vi "ImageInitRe.vi"(0 "Image in":refnum<class "Image.lvclass">, 11 "error in (no error)":errorcluster) -> (4 "Image out":refnum<class "Image.lvclass">, 15 "error out":errorcluster)   [LabVIEW 2012, in "Image.lvclass"]
uses:
  classes/Image.lvclass
  classes/Image.lvclass/Image.ctl
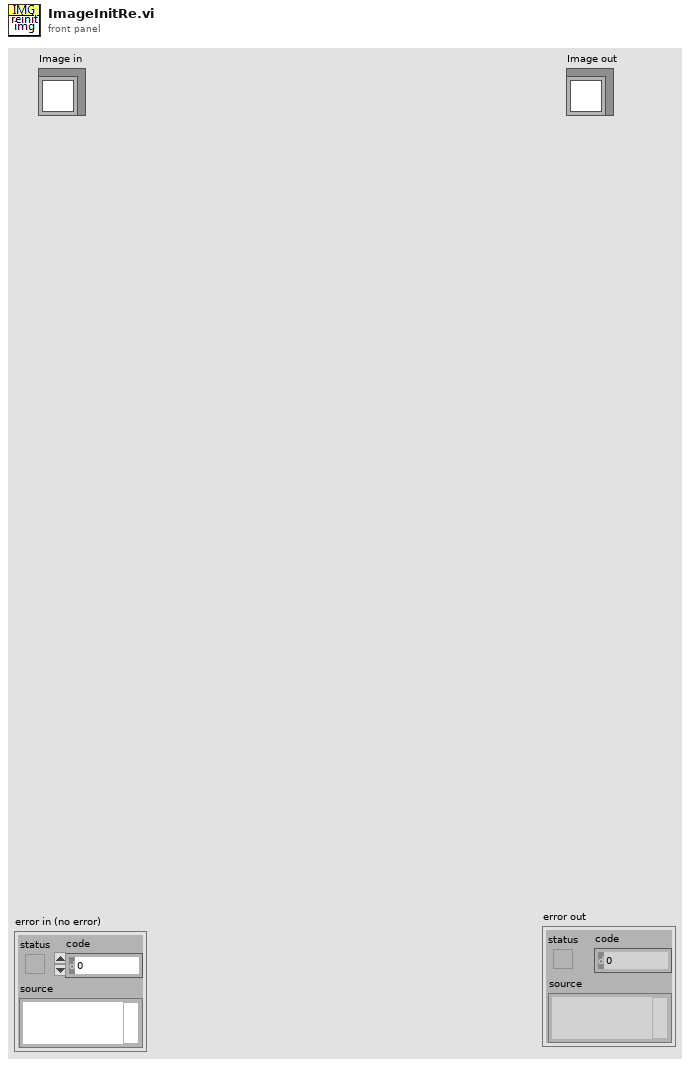
[diagram p1: front panel]
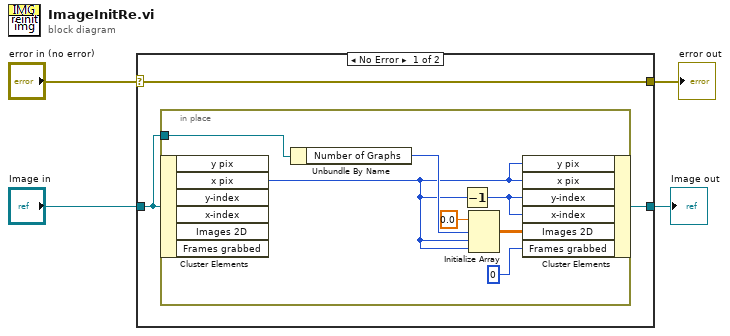
[diagram p0: block diagram]
diagram:
  n1 = case shown="No Error" "error in (no error)" {
    selector: "error in (no error)" -> [w7 w16]
    tunnel: [w7 w16] -> w3
    tunnel: [w5 w15] -> w1
    tunnel: "Image in" -> [w6 w15]
    frame No Error {
      n2 = in-place {
        in-place-border: w6 -> [w11]
        n3 = in-place-cluster #1(w6) -> ("x pix"=w8:i32)  [unwired: 5 out]
        n4 = Unbundle By Name(w11) -> ("Number of Graphs"=w10:i16)
        n5 = Decrement(x=w8) -> (x-1=w14:i32)
        n6 = Initialize Array(0.0 ("element"), w10, w8, w8) -> (w12:dbl[][][])
        n7 = in-place-cluster #1("y pix"=w8, "x pix"=w8, "y-index"=w14, "x-index"=w14, "Images 2D"=w12, "Frames grabbed"=0) -> (w5:refnum<class "Image.lvclass">)
      }
    }
    frame Error {
    }
  }
  "error out" <- w3
  "Image out" <- w1
